vi "mainRecord.vi"() -> ()   [LabVIEW 2017]
uses:
  globalUtilities.vi
  globalDevices.vi
  getComputerName.vi
panel:
  in  "hamamatsuReadoutSpeed":dbl=2.0
  in  "piezoEtlClockLock":bool
  in  "max (dpt)":dbl
  in  "min (dpt)":dbl
  in  "minmax":bool
  out "hamamatsuFrameAllocated":bool
  in  "stop":bool
  in  "volume height (um)":dbl=30.0 min=0.0 max=40.0
  in  "volumes per second":dbl=2.0
  out "folder name":string
  in  "frames per second":dbl=50.0
  # "SETTINGS"
  # "etl set on sensor mode in its GUI"
  # "2 vol/s etlSamplingRate = 5000\netlLatencyShift = 250"
  # "DIAGNOSTICS"
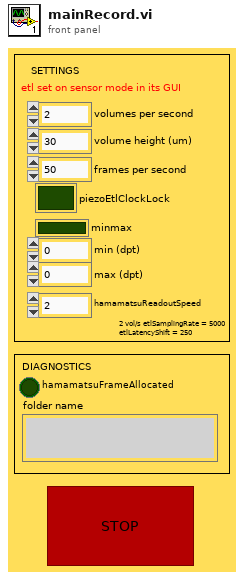
[diagram p1: front panel]
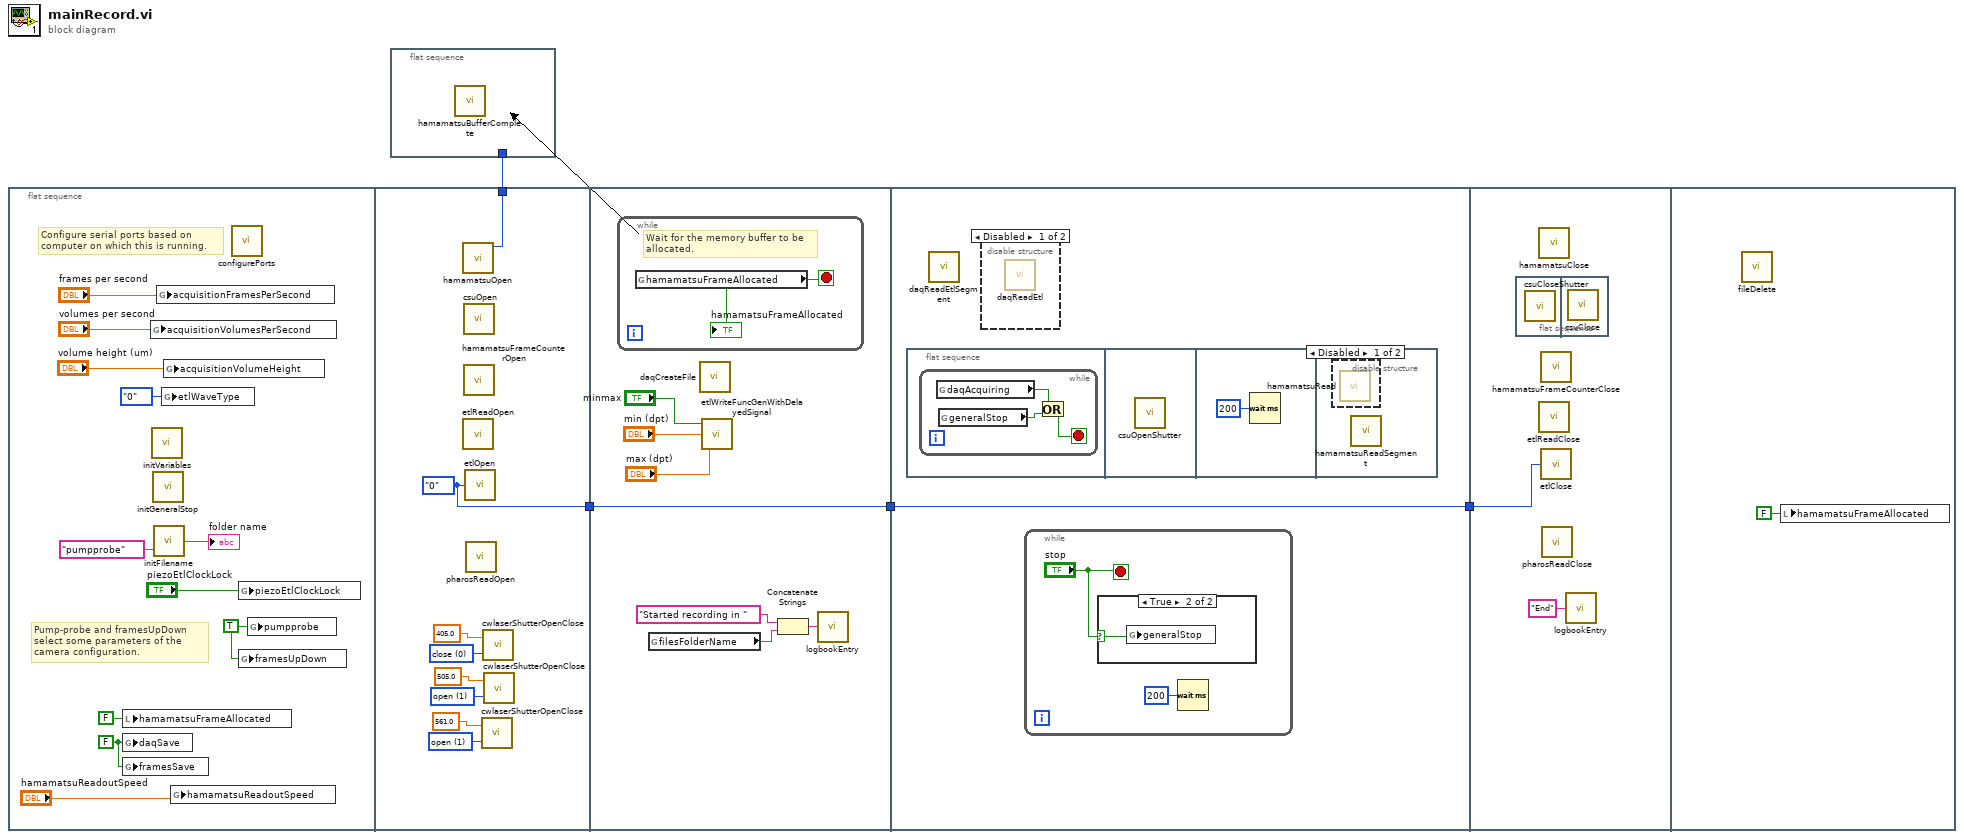
[diagram p0: block diagram]
diagram:
  n1 = flat-sequence {
    tunnel: [w23] -> w4
    tunnel: [w22] -> w1
    tunnel: [w30] -> w2
    tunnel: w1 -> [w30]
    tunnel: [w32] -> w3
    tunnel: w2 -> [w32]
    tunnel: w3 -> [w41]
    frame #0 {
      w7 = TRUE ("pumpprobe")
      w10 = FALSE ("daqSave")
      # "Pump-probe and framesUpDown \nselect some parameters of the \ncamera configuration."
      # "Configure serial ports based on\ncomputer on which this is running."
      n2 = local write "hamamatsuFrameAllocated"(FALSE ("hamamatsuFrameAllocated")) -> ()
      n3 = global write "globalUtilities.vi" "daqSave"(w10) -> ()
      n4 = global write "globalUtilities.vi" "framesSave"(w10) -> ()
      n5 = global write "globalUtilities.vi" "acquisitionVolumesPerSecond"("volumes per second") -> ()
      n6 = call "initVariables.vi"() -> ()  [unwired: 12 in]
      n7 = call "initGeneralStop.vi"() -> ()  [unwired: 1 in]
      n8 = call "initFilename.vi"("Experiment type"="pumpprobe") -> ("folder name"=→"folder name":string)  [unwired: 1 in]
      n9 = global write "globalUtilities.vi" "acquisitionFramesPerSecond"("frames per second") -> ()
      n10 = global write "globalDevices.vi" "etlWaveType"(enum16{"0", "1"}."0" ("etlWaveType")) -> ()
      n11 = global write "globalUtilities.vi" "acquisitionVolumeHeight"("volume height (um)") -> ()
      n12 = global write "globalDevices.vi" "hamamatsuReadoutSpeed"("hamamatsuReadoutSpeed") -> ()
      n13 = call "configurePorts.vi"() -> ()  [unwired: 12 in]
      n14 = global write "globalUtilities.vi" "piezoEtlClockLock"("piezoEtlClockLock") -> ()
      n15 = global write "globalUtilities.vi" "framesUpDown"(w7) -> ()
      n16 = global write "globalUtilities.vi" "pumpprobe"(w7) -> ()
    }
    frame #1 {
      w21 = u16 1 items=["close", "open"] ("mode")
      w19 = u16 1 items=["close", "open"] ("mode")
      w17 = u16 0 items=["close", "open"] ("mode")
      w22 = enum16{"0", "1"}."0" ("lens")
      n17 = call "hamamatsuOpen.vi"() -> ("Handle out"=w23:u32)  [unwired: 3 out]
      n18 = call "etlReadOpen.vi"() -> ()  [unwired: 2 in]
      n19 = call "csuOpen.vi"() -> ()  [unwired: 14 in, 2 out]
      n20 = call "hamamatsuFrameCounterOpen.vi"() -> ()  [unwired: 12 in]
      n21 = call "etlOpen.vi"("lens"=w22) -> ()  [unwired: 1 in]
      n22 = call "pharosReadOpen.vi"() -> ()  [unwired: 12 in]
      n23 = call "cwlaserShutterOpenClose.vi"("mode"=w21, "wavelength (nm)"=561.0) -> ()  [unwired: 1 out]
      n24 = call "cwlaserShutterOpenClose.vi"("mode"=w17, "wavelength (nm)"=405.0) -> ()  [unwired: 1 out]
      n25 = call "cwlaserShutterOpenClose.vi"("mode"=w19, "wavelength (nm)"=505.0) -> ()  [unwired: 1 out]
    }
    frame #2 {
      n26 = while {
        stop <- w31 stop-if-true
        # "Wait for the memory buffer to be\nallocated."
        n27 = global read "globalDevices.vi" "hamamatsuFrameAllocated"() -> (w31:bool)
        "hamamatsuFrameAllocated" <- w31
      }
      n28 = global read "globalUtilities.vi" "filesFolderName"() -> (w26:string)
      n29 = call "daqCreateFile.vi"() -> ()  [unwired: 12 in]
      n30 = call "etlWriteFuncGenWithDelayedSignal.vi"("max (dpt)"="max (dpt)", "min (dpt)"="min (dpt)", "minmax"="minmax") -> ()  [unwired: 1 in]
      n31 = Concatenate Strings("Started recording in ", w26) -> (w25:string)
      n32 = call "logbookEntry.vi"("Log book entry"=w25) -> ()  [unwired: 2 out]
    }
    frame #3 {
      n33 = flat-sequence {
        frame #0 {
          n34 = while {
            stop <- w38 stop-if-true
            n35 = global read "globalUtilities.vi" "daqAcquiring"() -> (w37:bool)
            n36 = global read "globalUtilities.vi" "generalStop"() -> (w36:bool)
            n37 = Or(x=w37, y=w36) -> (x .or. y?=w38:bool)
          }
        }
        frame #1 {
          n38 = call "csuOpenShutter.vi"() -> ()  [unwired: 16 in]
        }
        frame #2 {
          n39 = Wait (ms)(milliseconds to wait=u32 200) -> ()  [unwired: 1 out]
        }
        frame #3 {
          n40 = disable-structure shown="Disabled" {
            frame Disabled {
              n41 = call "hamamatsuRead.vi"() -> ()  [unwired: 12 in]
            }
            frame Enabled {
            }
          }
          n42 = call "hamamatsuReadSegment.vi"() -> ()  [unwired: 12 in]
        }
      }
      n43 = call "daqReadEtlSegment.vi"() -> ()  [unwired: 3 in]
      n44 = disable-structure shown="Disabled" {
        frame Disabled {
          n45 = call "daqReadEtl.vi"() -> ()  [unwired: 3 in]
        }
        frame Enabled {
        }
      }
      n46 = while {
        stop <- "stop" stop-if-true
        n47 = case shown="True" "stop" {
          selector: "stop" -> [_ w35]
          frame False {
          }
          frame True {
            n48 = global write "globalUtilities.vi" "generalStop"(w35) -> ()
          }
        }
        n49 = Wait (ms)(milliseconds to wait=u32 200) -> ()  [unwired: 1 out]
      }
    }
    frame #4 {
      n50 = flat-sequence {
        frame #0 {
          n51 = call "csuCloseShutter.vi"() -> ()  [unwired: 16 in]
        }
        frame #1 {
          n52 = call "csuClose.vi"() -> ()  [unwired: 12 in]
        }
      }
      n53 = call "hamamatsuClose.vi"() -> ()  [unwired: 1 out]
      n54 = call "etlReadClose.vi"() -> ()  [unwired: 12 in]
      n55 = call "hamamatsuFrameCounterClose.vi"() -> ()  [unwired: 12 in]
      n56 = call "etlClose.vi"("lens"=w41) -> ()  [unwired: 1 in]
      n57 = call "pharosReadClose.vi"() -> ()  [unwired: 12 in]
      n58 = call "logbookEntry.vi"("Log book entry"="End") -> ()  [unwired: 2 out]
    }
    frame #5 {
      n59 = call "fileDelete.vi"() -> ()  [unwired: 12 in]
      n60 = local write "hamamatsuFrameAllocated"(FALSE ("hamamatsuFrameAllocated")) -> ()
    }
  }
  n61 = flat-sequence {
    tunnel: w4 -> [_]
    frame #0 {
      n62 = call "hamamatsuBufferComplete.vi"() -> ()  [unwired: 12 in]
    }
  }
